vi "Read File Path.vi"(4 "Error In":errorcluster, 7 "Text In":refnum<class "Config Data_Text.lvclass">) -> (0 "Error Out":errorcluster, 2 "File Path":path, 3 "Text Out":refnum<class "Config Data_Text.lvclass">)   [LabVIEW 2014, in "Config Data.lvlib" / "Config Data_Text.lvclass"]
uses:
  Config Data_Text.lvclass
  Config Data_Text.lvclass/Config Data_Text.ctl
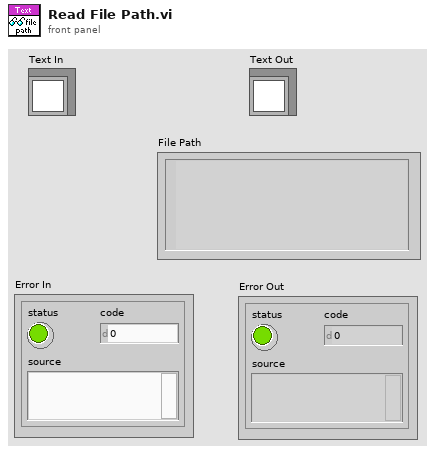
[diagram p1: front panel]
types:
  T1 = typedef "Config Data.lvlib/Config Data_Text.lvclass/Text Data.ctl" = cluster{"File Path":path}
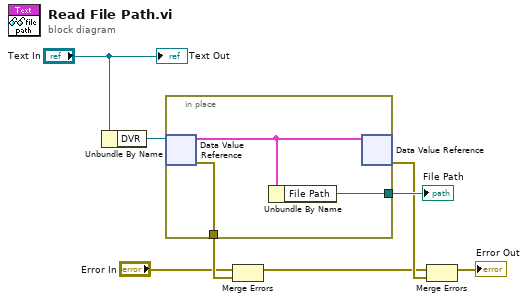
[diagram p0: block diagram]
diagram:
  n1 = Unbundle By Name("Text In") -> ("DVR"=w7:refnum<data-value>)
  n2 = in-place {
    in-place-border: [w11] -> w6
    in-place-border: [w9] -> w5
    n3 = in-place-dvr #1(w7) -> (w10:T1, w9:errorcluster)
    n4 = Unbundle By Name(w10) -> ("File Path"=w11:path)
    n5 = in-place-dvr #1(w10) -> (w3:errorcluster)  [unwired: 1 out]
  }
  "File Path" <- w6
  n6 = Merge Errors("Error In", w5) -> (w2:errorcluster)
  n7 = Merge Errors(w2, w3) -> (→"Error Out":errorcluster)
  "Text Out" <- "Text In"
